vi "4461 - Create IO Channels Parallel Uneven - SINGLE TASK.vi"(6 "error in":errorcluster, 7 "Sampling Stuff (AI & AO)":T3={"sampling info (DAQ class)"={"Fs"=0.0, "#s"=0.0}, "sample mode (DAQ class)"=10178, "AI Buffer Size (S)"=10} {"sample mode (DAQ class)" items=["Finite Samples"=10178, "Continuous Samples"=10123]}) -> (2 "AO Task":refnum<k21>, 3 "AI Task":refnum<k21>, 4 "error out":errorcluster)   [LabVIEW 2016]
uses:
  <vilib>/DAQmx/write.llb/DAQmx Write (Analog 1D Wfm NChan NSamp).vi
  <vilib>/DAQmx/read.llb/DAQmx Read (Analog 1D Wfm NChan NSamp).vi
  <vilib>/DAQmx/create/channels.llb/DAQmx Create Channel (AI-Voltage-Basic).vi
  <vilib>/DAQmx/configure/timing.llb/DAQmx Timing (Sample Clock).vi
  <vilib>/DAQmx/create/channels.llb/DAQmx Create Channel (AO-Voltage-Basic).vi
  <vilib>/DAQmx/configure/trigger.llb/DAQmx Start Trigger (Digital Edge).vi
  <vilib>/DAQmx/miscellaneous.llb/DAQmx Fill In Error Info.vi
  <resource>/objmgr/daqmx.rc
panel:
  in  "SyncPulse.SyncTime":dbl
  in  "RefClk.Src":tag
  in  "AO Configuration":T1={"AO Channels (DAQ class)"="", "minimum value"=-10.0, "maximum value"=10.0, "output terminal configuration"=-1} {"output terminal configuration" items=["Default"=-1, "RSE"=10083, "Differential"=10106, "Pseudodifferential"=12529]; "maximum value" format="%0.2f"; "minimum value" format="%0.2f"}
  in  "AI Configuration":T2={"AI Channels (DAQ class)"="", "minimum value (DAQ(?))"=-5.0, "maximum value (DAQ(?))"=5.0, "AI.Coupling (DAQmx)"=10045, "input terminal configuration (DAQmx)"=-1} {"input terminal configuration (DAQmx)" items=["default"=-1, "RSE"=10083, "NRSE"=10078, "Differential"=10106, "Pseudodifferential"=12529]; "AI.Coupling (DAQmx)" items=["AC"=10045, "DC"=10050, "GND"=10066]; "maximum value (DAQ(?))" format="%0.2f"; "minimum value (DAQ(?))" format="%0.2f"}
  in  "AO Array":waveform(dbl)[](array[waveform])
  out "AI.FilterDelay":dbl
  out "AI.Gain":dbl
  # "AI and AO CONFIG"
  # "OUTPUTS"
  # "INPUTS"
  # "These are just for debugging / monitoring"
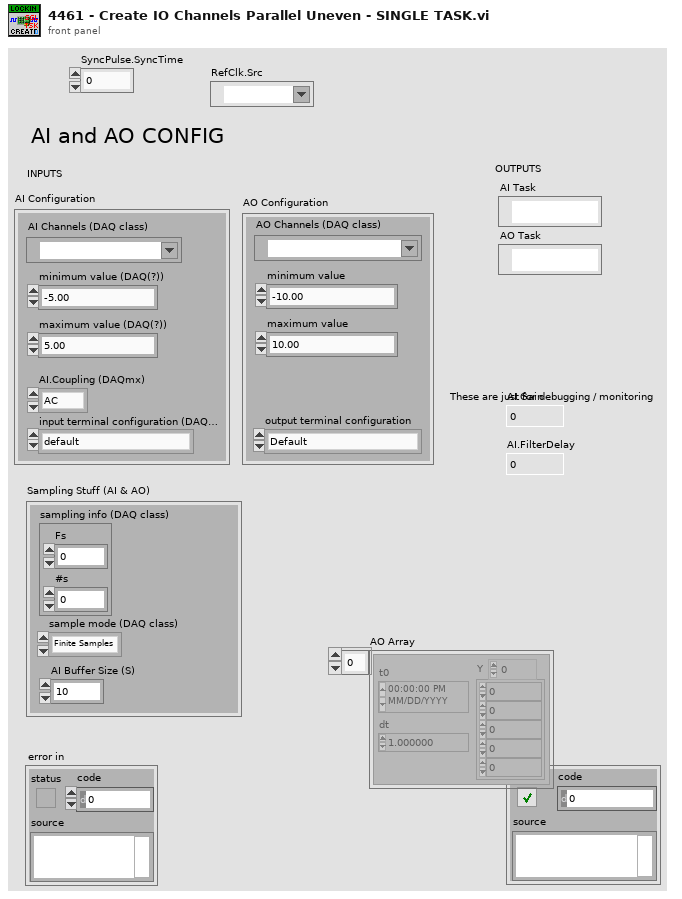
[diagram p1: front panel]
types:
  T1 = cluster{"AO Channels (DAQ class)":tag, "minimum value":dbl, "maximum value":dbl, "output terminal configuration":i32}
  T2 = cluster{"AI Channels (DAQ class)":tag, "minimum value (DAQ(?))":dbl, "maximum value (DAQ(?))":dbl, "AI.Coupling (DAQmx)":i32, "input terminal configuration (DAQmx)":i32}
  T3 = cluster{"sampling info (DAQ class)":cluster{"Fs":dbl, "#s":dbl}, "sample mode (DAQ class)":i32, "AI Buffer Size (S)":i32}
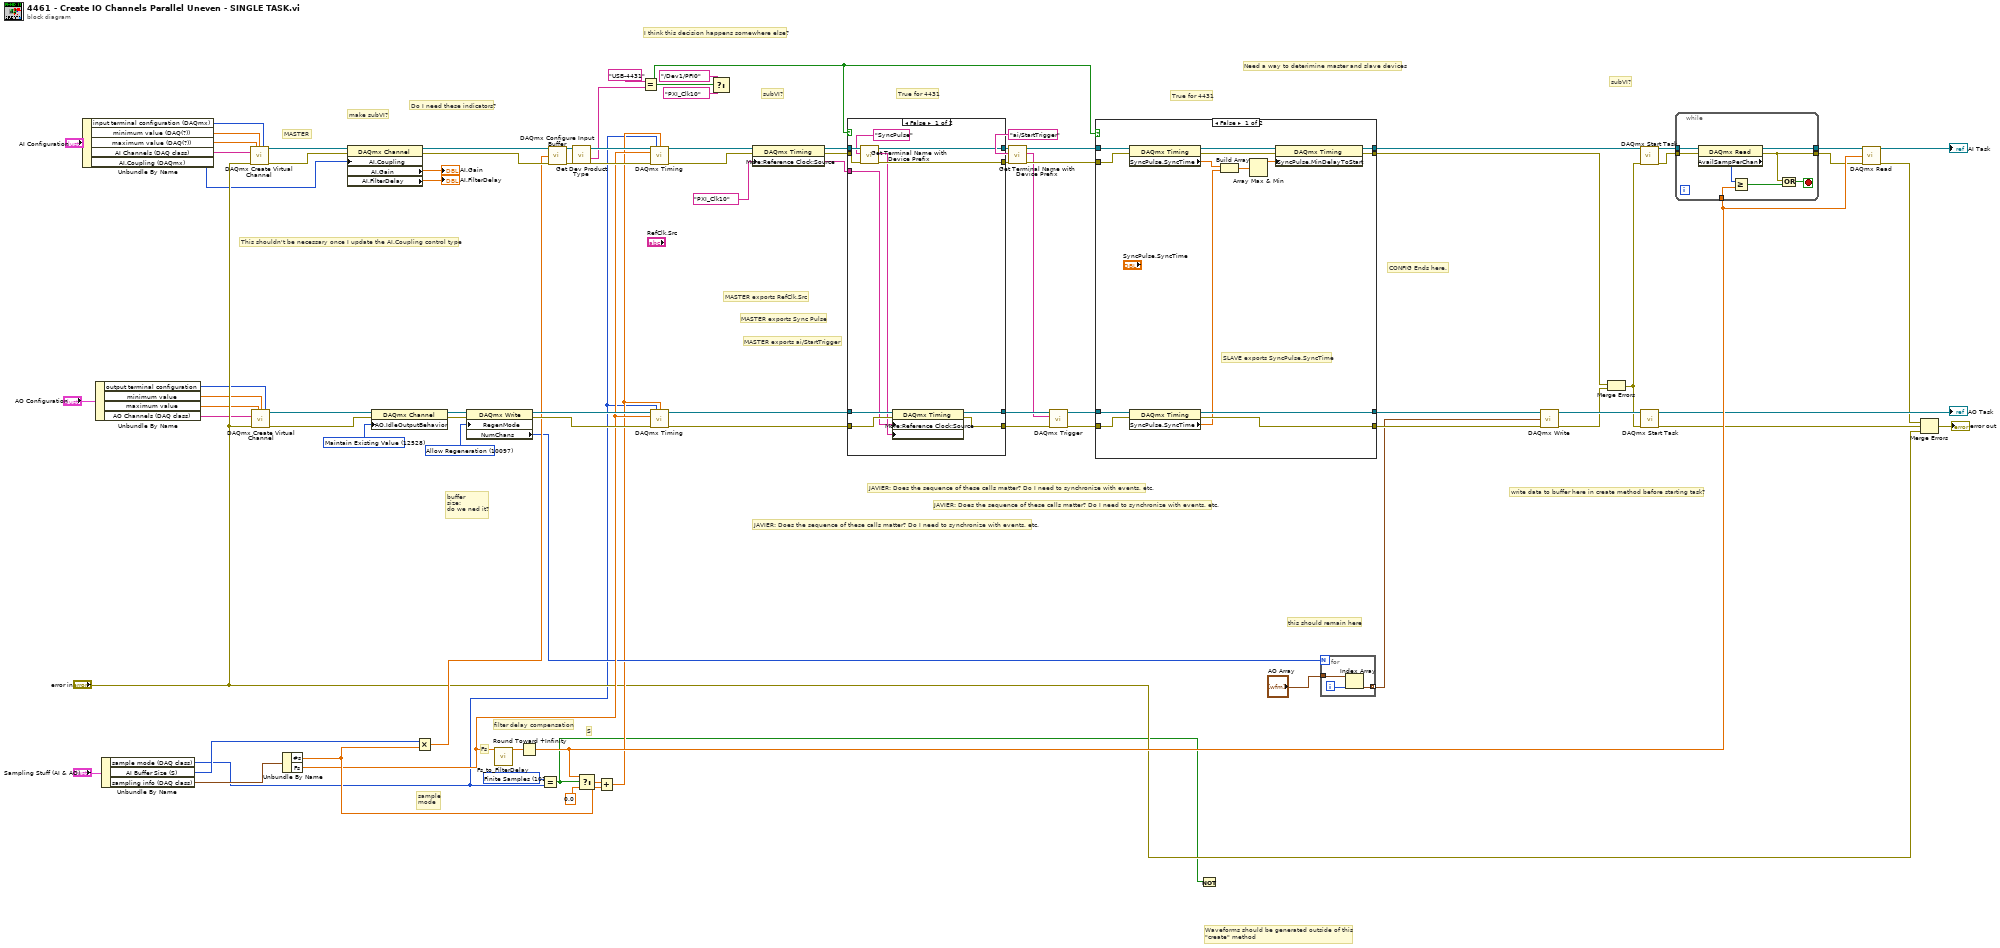
[diagram p0: block diagram]
diagram:
  w1 = tag "PXI_Clk10" ("RefClk.Src")
  w78 = 10097 items=["Allow Regeneration"=10097, "Do Not Allow Regeneration"=10158] ("RegenMode")
  w80 = 12528 items=["Zero Volts"=12526, "High-Impedance"=12527, "Maintain Existing Value"=12528] ("AO.IdleOutputBehavior")
  w81 = 10178 items=["Finite Samples"=10178, "Continuous Samples"=10123] ("sample mode 2")
  # "CONFIG Ends here."
  # "Need a way to deterimine master and slave devices"
  # "JAVIER: Does the sequence of these calls matter? Do I need to synchronize with events, etc."
  # "JAVIER: Does the sequence of these calls matter? Do I need to synchronize with events, etc."
  # "filter delay compensation"
  # "subVI?"
  # "JAVIER: Does the sequence of these calls matter? Do I need to synchronize with events, etc."
  # "MASTER exports ai/StartTrigger"
  # "MASTER exports Sync Pulse"
  # "MASTER exports RefClk.Src"
  # "subVI?"
  # "I think this decision happens somewhere else?"
  # "make subVI?"
  # "Do I need these indicators?"
  # "write data to buffer here in create method before starting task?"
  # "this should remain here"
  # "True for 4431"
  # "True for 4431"
  # "Waveforms should be generated outside of this \n\"create\" method"
  # "This shouldn't be necessary once I update the AI.Coupling control type"
  # "MASTER"
  # "S"
  # "Fs"
  # "sample\nmode"
  # "buffer\nsize:\ndo we ned it?"
  n1 = Unbundle By Name("AI Configuration") -> ("input terminal configuration (DAQmx)"=w9:i32, "minimum value (DAQ(?))"=w10:dbl, "maximum value (DAQ(?))"=w11:dbl, "AI Channels (DAQ class)"=w12:tag, "AI.Coupling (DAQmx)"=w3:i32)
  n2 = Unbundle By Name("AO Configuration") -> ("output terminal configuration"=w7:i32, "minimum value"=w6:dbl, "maximum value"=w5:dbl, "AO Channels (DAQ class)"=w4:tag)
  n3 = Unbundle By Name("Sampling Stuff (AI & AO)") -> ("sample mode (DAQ class)"=w14:i32, "AI Buffer Size (S)"=w15:i32, "sampling info (DAQ class)"=w16:cluster{"Fs":dbl, "#s":dbl})
  n4 = call-poly <vilib>:"DAQmx Create Virtual Channel.vi"("maximum value"=w11, "minimum value"=w10, "input terminal configuration"=w9, "physical channels"=w12, "error in"="error in") -> ("task out"=w38:refnum<k21>, "error out"=w37:errorcluster)  [unwired: 9 in]
  n5 = call-poly <vilib>:"DAQmx Create Virtual Channel.vi"("maximum value"=w5, "minimum value"=w6, "output terminal configuration"=w7, "physical channels"=w4, "error in"="error in") -> ("task out"=w36:refnum<k21>, "error out"=w35:errorcluster)  [unwired: 9 in]
  n6 = Unbundle By Name(w16) -> ("#s"=w79:dbl, "Fs"=w40:dbl)
  n7 = property class="DAQmx Channel"(reference=w38, error in=w37, "AI.Coupling"=w3) -> (reference out=w53:refnum<k21>, error out=w52:errorcluster, "AI.Gain"=→"AI.Gain":dbl, "AI.FilterDelay"=→"AI.FilterDelay":dbl)
  n8 = property class="DAQmx Channel"(reference=w36, error in=w35, "AO.IdleOutputBehavior"=w80) -> (reference out=w34:refnum<k21>, error out=w33:errorcluster)
  n9 = Multiply(x=w15, y=w79) -> (x*y=w39:dbl)
  n10 = property class="DAQmx Write"(reference=w34, error in=w33, "RegenMode"=w78) -> (reference out=w60:refnum<k21>, error out=w58:errorcluster, "NumChans"=w27:u32)
  n11 = call "Fs_to_FilterDelay.vi"("Fs"=w40) -> ("Total Filter Delay (samples)"=w84:dbl)  [unwired: 10 in]
  n12 = Round Toward +Infinity(x=w84) -> (ceil(x): smallest int >= x=w77:dbl)
  n13 = Equal?(x=w81, y=w14) -> (x = y?=w21:bool)
  n14 = call <vilib>:"DAQmx Configure Input Buffer.vi"("task/channels in"=w53, "buffer size (in samples per channel)"=w39, "error in"=w52) -> ("task out"=w32:refnum<k21>, "error out"=w31:errorcluster)  [unwired: 11 in]
  n15 = call "Get Dev Product Type.vi"("error in (no error)"=w31, "Refnum in"=w32) -> ("error out"=w47:errorcluster, "ProductType"=w44:string, "Refnum out"=w46:refnum<k21>)  [unwired: 7 in]
  n16 = Select(t=w77, s=w21, f=0.0) -> (s? t:f=w82:dbl)
  n17 = Add(x=w82, y=w79) -> (x+y=w23:dbl)
  n18 = Equal?(x="USB-4431" ("ProductType"), y=w44) -> (x = y?=w41:bool)
  n19 = call-poly <vilib>:"DAQmx Timing.vi"("task/channels in"=w46, "sample mode"=w14, "samples per channel"=w23, "rate"=w40, "error in"=w47) -> ("task out"=w75:refnum<k21>, "error out"=w69:errorcluster)  [unwired: 9 in]
  n20 = call-poly <vilib>:"DAQmx Timing.vi"("task/channels in"=w60, "sample mode"=w14, "samples per channel"=w23, "rate"=w40, "error in"=w58) -> ("task out"=w59:refnum<k21>, "error out"=w42:errorcluster)  [unwired: 9 in]
  n21 = Select(t=tag "/Dev1/PFI0" ("RefClk.Src"), s=w41, f=tag "PXI_Clk10" ("RefClk.Src")) -> ()  [unwired: 1 out]
  n22 = property class="DAQmx Timing"(reference=w75, error in=w69, "More:Reference Clock:Source"=w1) -> (reference out=w61:refnum<k21>, error out=w43:errorcluster)
  n23 = case shown="False" w41 {
    tunnel: [w96 w100] -> w74
    tunnel: [w95 w99] -> w73
    tunnel: [w94 w98] -> w68
    tunnel: [w93 w97] -> w67
    tunnel: w61 -> [w92 w100]
    tunnel: w59 -> [w91 w98]
    tunnel: w43 -> [w87 w99]
    tunnel: w1 -> [w86 _]
    tunnel: w42 -> [w90 w97]
    frame False {
      n24 = call "Get Terminal Name with Device Prefix.vi"("error in (no error)"=w87, "Local Terminal Name"="SyncPulse", "task/channels in"=w92) -> ("error out"=w95:errorcluster, "Terminal Name with Device Prefix"=w88:tag, "task out"=w96:refnum<k21>)  [unwired: 6 in]
      n25 = property class="DAQmx Timing"(reference=w91, error in=w90, "More:Reference Clock:Source"=w86, "More:Synchronization Pulse:Source"=w88) -> (reference out=w94:refnum<k21>, error out=w93:errorcluster)
    }
    frame True {
    }
  }
  n26 = call "Get Terminal Name with Device Prefix.vi"("error in (no error)"=w73, "Local Terminal Name"="ai/StartTrigger", "task/channels in"=w74) -> ("error out"=w71:errorcluster, "Terminal Name with Device Prefix"=w64:tag, "task out"=w72:refnum<k21>)  [unwired: 6 in]
  n27 = call-poly <vilib>:"DAQmx Trigger.vi"("task/channels in"=w68, "source"=w64, "error in"=w67) -> ("task out"=w66:refnum<k21>, "error out"=w65:errorcluster)  [unwired: 11 in]
  n28 = case shown="False" w41 {
    tunnel: w72 -> [w114 w118]
    tunnel: w71 -> [w113 w117]
    tunnel: [w112 w117] -> w18
    tunnel: [w111 w118] -> w70
    tunnel: w66 -> [w110 w116]
    tunnel: w65 -> [w109 w115]
    tunnel: [w108 w116] -> w63
    tunnel: [w107 w115] -> w62
    frame False {
      # "SLAVE exports SyncPulse.SyncTime"
      n29 = property class="DAQmx Timing"(reference=w114, error in=w113) -> (reference out=w104:refnum<k21>, error out=w105:errorcluster, "SyncPulse.SyncTime"=w106:dbl)
      n30 = property class="DAQmx Timing"(reference=w110, error in=w109) -> (reference out=w108:refnum<k21>, error out=w107:errorcluster, "SyncPulse.SyncTime"=w101:dbl)
      n31 = Build Array(w106, w101) -> (w103:dbl[])
      n32 = Array Max & Min(array=w103) -> (max value=w102:dbl)  [unwired: 3 out]
      n33 = property class="DAQmx Timing"(reference=w104, error in=w105, "SyncPulse.MinDelayToStart"=w102) -> (reference out=w111:refnum<k21>, error out=w112:errorcluster)
    }
    frame True {
    }
  }
  n34 = Not(x=w21) -> ()  [unwired: 1 out]
  n35 = for {
    N: w27 -> [_]
    tunnel: [w119] -> w28 mode=indexing
    tunnel: "AO Array" -> [w120]
    i -> [w121]
    n36 = Index Array(array=w120, index=w121) -> (element=w119:waveform(dbl))
  }
  n37 = call-poly <vilib>:"DAQmx Write.vi"("task/channels in"=w63, "data"=w28, "error in"=w62) -> ("task out"=w76:refnum<k21>, "error out"=w20:errorcluster)  [unwired: 10 in, 1 out]
  n38 = Merge Errors(w18, w20) -> (w19:errorcluster)
  n39 = call <vilib>:"DAQmx Start Task.vi"("task/channels in"=w70, "error in"=w19) -> ("task out"=w56:refnum<k21>, "error out"=w49:errorcluster)  [unwired: 12 in]
  n40 = call <vilib>:"DAQmx Start Task.vi"("task/channels in"=w76, "error in"=w19) -> ("task out"=→"AO Task":refnum<k21>, "error out"=w54:errorcluster)  [unwired: 12 in]
  n41 = while {
    tunnel: w56 -> [w129]
    tunnel: w49 -> [w128]
    tunnel: [w124] -> w55
    tunnel: [w127] -> w57
    tunnel: w77 -> [w126]
    stop <- w125 stop-if-true
    n42 = property class="DAQmx Read"(reference=w129, error in=w128) -> (reference out=w127:refnum<k21>, error out=w124:errorcluster, "AvailSampPerChan"=w123:u32)
    n43 = Greater Or Equal?(x=w123, y=w126) -> (x >= y?=w122:bool)
    n44 = Compound Arithmetic op=OR(w124, w122) -> (w125:bool)
  }
  n45 = call-poly <vilib>:"DAQmx Read.vi"("task/channels in"=w57, "number of samples per channel"=w77, "error in"=w55) -> ("task out"=→"AI Task":refnum<k21>, "error out"=w25:errorcluster)  [unwired: 10 in, 1 out]
  n46 = Merge Errors(w25, w54, "error in") -> (→"error out":errorcluster)
